vi "IMUOpen.vi"(4 "MagCal":bool, 5 "Accel Set":T5={"Data Rate"=enum."1.344 kHz", "Range"=0, "HPF Enable"=FALSE, "HPCF"=enum."00", "Sense Enable"=TRUE, "Accel Scale"={"Xscale"=1.0, "Yscale"=1.0, "Zscale"=1.0}, "Motion Thresh"=0.0} {"Range" items=["+/- 2 G", "+/- 4 G", "+/- 8 G", "+/- 16 G"]}, 6 "Mag Set":T2={"Data Rate"=enum."220 Hz", "Range"=1, "Sense Enable"=TRUE, "Mag Scale"={"Xscale"=1.0, "Yscale"=1.00987, "Zscale"=1.0}, "Mag Offset"={"Xzero"=0.181818, "Yzero"=-0.642644, "Zzero"=0.0}, "Anomaly Thresh"=0.646769, "Local Mag"=27.7309} {"Range" items=["+/- 130 uT"=1, "+/- 190 uT"=2, "+/- 250 uT"=3, "+/- 400 uT"=4, "+/- 470 uT"=5, "+/- 560 uT"=6, "+/- 810 uT"=7]}, 7 "Gyro Set":T6={"Data Rate"=enum."800 Hz", "Range"=0, "HPF Enable"=FALSE, "HPCF"=enum."0000", "Sense Enable"=TRUE} {"Range" items=["+/- 245 deg/sec", "+/- 500 deg/sec", "+/- 2000 deg/sec"]}, 8 "error in (no error)":errorcluster, 9 "Fast":bool=TRUE, 10 "CalSamples":i32=60, 11 "I2C Bus":T4) -> (0 "error out":errorcluster, 2 "Cal Result":T1, 3 "AdaIMUDevRef Out":T7={"DevStatus"={"status"=FALSE, "code"=0, "source"=""}, "Gyro Address"=0, "Gyro Range"=0, "Mean Rates"={"Xmo"=0.0, "Ymo"=0.0, "Zmo"=0.0}, "StdDev Rates"={"Xsdo"=0.0, "Ysdo"=0.0, "Zsdo"=0.0}, "Fast"=FALSE, "Reset"=FALSE, "Accel Address"=0, "Accel Range"=0, "Accel Scale"={"Xscale"=0.0, "Yscale"=0.0, "Zscale"=0.0}, "Mag Address"=0, "Mag Range"=0, "G Sense"=FALSE, "A Sense"=FALSE, "M Sense"=FALSE, "Accel Offset"={"Xzero"=0.0, "Yzero"=0.0, "Zzero"=0.0}, "Motion Thresh"=0.0, "Mag Scale"={"Xscale"=1.0, "Yscale"=1.0, "Zscale"=1.0}, "Mag Offset"={"Xzero"=1.0, "Yzero"=1.0, "Zzero"=1.0}, "I2C Bus"=enum."I2C On-Board", "Handle"=0, "Controller"=enum."Controller 1", "Anomaly Thresh"=0.0, "Local Mag"=0.0})   [LabVIEW 2014]
uses:
  IMUDevRef.ctl
  <vilib>/Rock Robotics/SystemInterfaces/i2clib/i2c_bus.ctl
  <vilib>/Rock Robotics/SystemInterfaces/Typedef/FPGA_TypedefDigitalModule.ctl
  <vilib>/Platform/TimedLoop/XDataNode/timing_clust.ctl
  <vilib>/Platform/TimedLoop/XDataNode/nitl_modes.ctl
  <vilib>/Platform/TimedLoop/XDataNode/wakeup.ctl
  <vilib>/Utility/file.llb/Write To Spreadsheet File (DBL).vi
  <vilib>/platform/TimedLoop/XDataNode/XDataNode.xnode
  <vilib>/Platform/TimedLoop/XDataNode/XDNodeRunTimeDep.lvlib
  <vilib>/Analysis/NI_AALBase.lvlib
panel:
  in  "Mag Set 2":T2={"Data Rate"=enum."220 Hz", "Range"=1, "Sense Enable"=TRUE, "Mag Scale"={"Xscale"=1.0, "Yscale"=1.0, "Zscale"=1.0}, "Mag Offset"={"Xzero"=0.0, "Yzero"=0.0, "Zzero"=0.0}, "Anomaly Thresh"=0.0, "Local Mag"=0.0} {"Range" items=["+/- 130 uT"=1, "+/- 190 uT"=2, "+/- 250 uT"=3, "+/- 400 uT"=4, "+/- 470 uT"=5, "+/- 560 uT"=6, "+/- 810 uT"=7]}
  out "XY Mag, Cal'd":cluster{dbl[], dbl[]}(graph)
  out "Anomaly Tol (uT)":dbl
  out "Local Magnitude (uT)":dbl
  out "Mid-Pnt":dbl
  out "Half-Range":dbl
  in  "Controller":T3
  out "Late?":bool
  in  "Period":i64=20
  out "Yaw":dbl(knob) scale=-180.0..180.0
  out "Pitch":dbl(knob) scale=-90.0..90.0
  out "Roll":dbl(knob) scale=-180.0..180.0
  in  "Reset":bool
  in  "Accel Set 2":T5={"Data Rate"=enum."1.344 kHz", "Range"=0, "HPF Enable"=FALSE, "HPCF"=enum."00", "Sense Enable"=TRUE, "Accel Scale"={"Xscale"=0.9852, "Yscale"=1.0101, "Zscale"=1.0101}, "Motion Thresh"=0.04} {"Range" items=["+/- 2 G", "+/- 4 G", "+/- 8 G", "+/- 16 G"]}
  in  "Gyro Set 2":T6={"Data Rate"=enum."800 Hz", "Range"=0, "HPF Enable"=FALSE, "HPCF"=enum."0000", "Sense Enable"=TRUE} {"Range" items=["+/- 245 deg/sec", "+/- 500 deg/sec", "+/- 2000 deg/sec"]}
  out "Xmagscale":dbl
  out "Ymagscale":dbl
  out "Ymagzero":dbl
  out "Xmagzero":dbl
  out "XY Mag":cluster{dbl[], dbl[]}(graph)
  out "stop loop":bool
  # "EXAMPLE MAGNETOMETER CAL PLOT - FOR REFERENCE"
  # "Magnetometer Cal Results"
  # "Use LM as Local Mag,\nwhich should be NOAA\nHorizontal Mag Intensity.\nUse AT as minimum\nAnomaly Threshold."
  # "Magnetometer Calibration Data Result\n\nLook for a constant radius circle - if not, repeat calibration.\n\nMagnetometer measurement error is generally classified into two categories, Hard Iron and Soft Iron effects.  Only Hard Iron effects\nare compensated here, as they appear more dominate.  Soft Iron effect compensation is a future improvement.  Performance is\nadequate as long as sources of Soft Iron distortion (non-magnetized Iron, Nickle, and Cobalt) are kept away from sensor\n(or vice versa).  If an ellipse is displayed, there is Soft Iron magnetic field interference.  Ensure the cal plot has equally sized X and Y\naxis ranges prior to visually inspecting the cal plot and making an ellipse determination.  If Soft Iron is detected, either relocate the\nIMU or discover and remove the offending material.  Run all motors and other actuators to verify that the Yaw output of the\nComplementary Filter is not significantly affected.  If so, it may be possible to relocate the IMU or shield the motor with\nmu-metal or similar.  Do not shield the IMU!"
  # "Reserved for future use."
  # "These controls/indicators are non-operational / they are here as example documentation only."
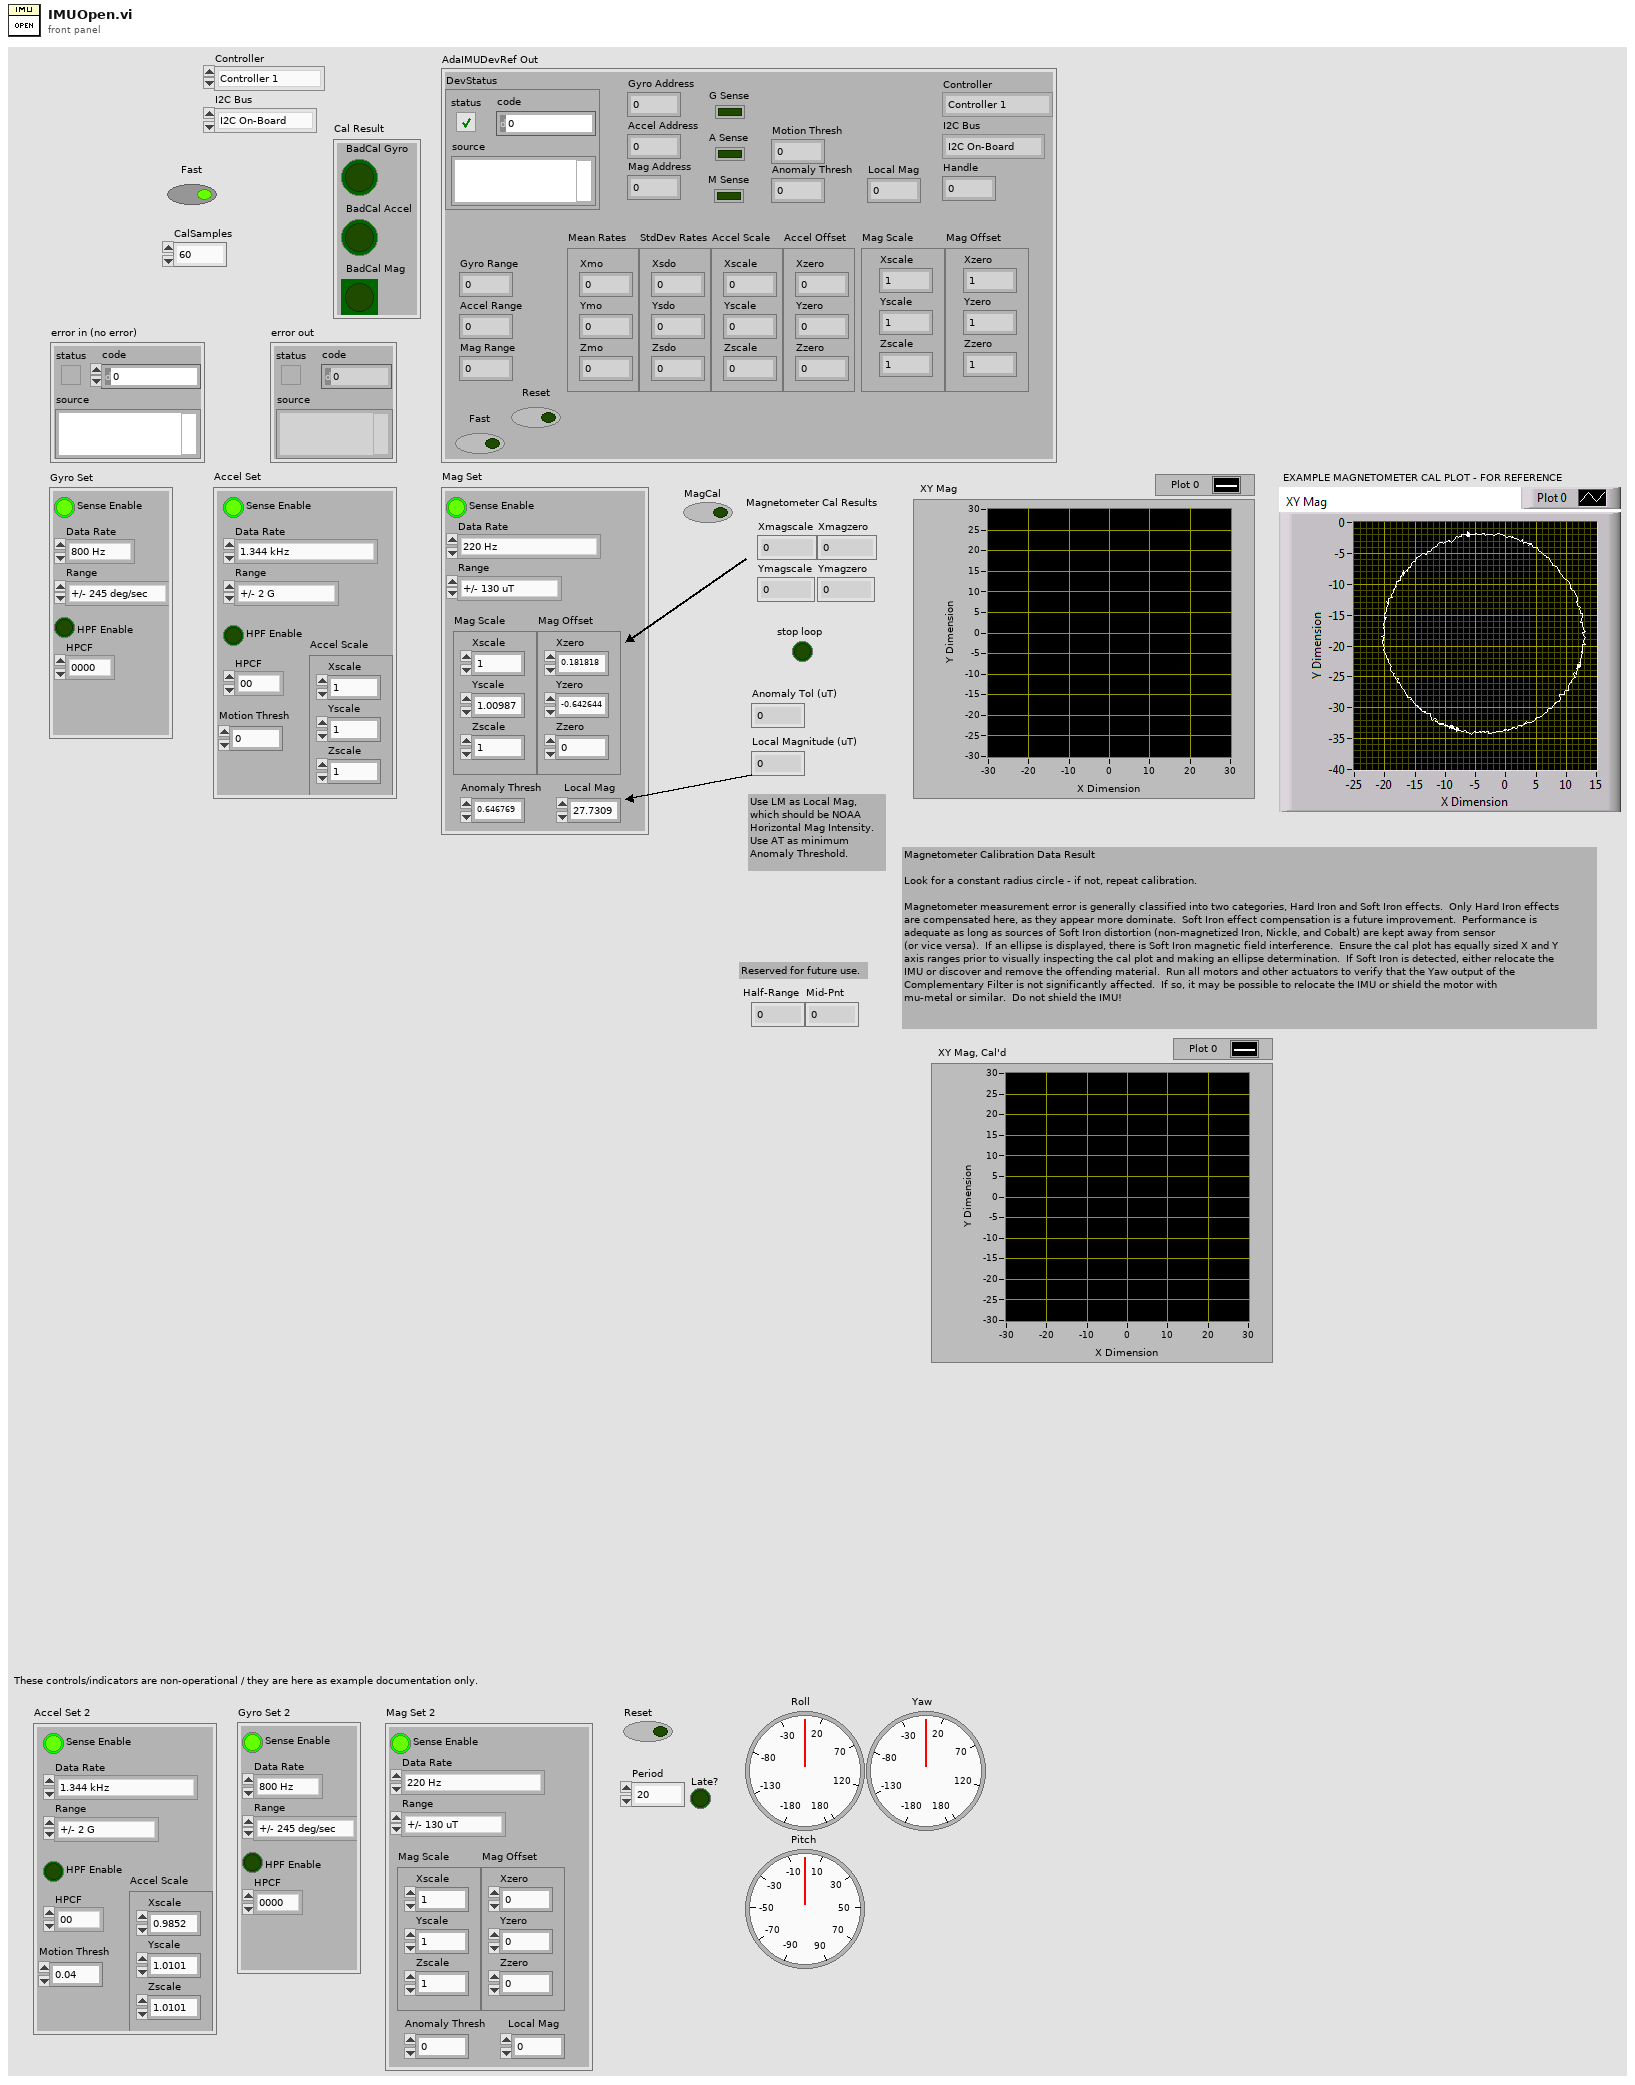
[diagram p1: front panel]
types:
  T1 = cluster{"BadCal Gyro":bool, "BadCal Accel":bool, "BadCal Mag":bool}
  T2 = cluster{"Data Rate":enum8{"0.75 Hz", "1.5 Hz", "3.0 Hz", "7.5 Hz", "15 Hz", "30 Hz", "75 Hz", "220 Hz"}, "Range":u8, "Sense Enable":bool, "Mag Scale":cluster{"Xscale":dbl, "Yscale":dbl, "Zscale":dbl}, "Mag Offset":cluster{"Xzero":dbl, "Yzero":dbl, "Zzero":dbl}, "Anomaly Thresh":dbl, "Local Mag":dbl}
  T3 = typedef "FPGA_TypedefDigitalModule.ctl" = enum16{"Controller 1"}
  T4 = typedef "i2c_bus.ctl" = enum16{"I2C On-Board", "I2C MXP", "Invalid"}
  T5 = cluster{"Data Rate":enum8{"Power-down mode", "1 Hz", "10 Hz", "25 Hz", "50 Hz", "100 Hz", "200 Hz", "400 Hz", "Low-power mode only", "1.344 kHz"}, "Range":u8, "HPF Enable":bool, "HPCF":enum8{"00", "01", "10", "11"}, "Sense Enable":bool, "Accel Scale":cluster{"Xscale":dbl, "Yscale":dbl, "Zscale":dbl}, "Motion Thresh":dbl}
  T6 = cluster{"Data Rate":enum8{"100 Hz", "200 Hz", "400 Hz", "800 Hz"}, "Range":u8, "HPF Enable":bool, "HPCF":enum8{"0000", "0001", "0010", "0011", "0100", "0101", "0110", "0111", "1000", "1001"}, "Sense Enable":bool}
  T7 = typedef "IMUDevRef.ctl" = cluster{"DevStatus":errorcluster, "Gyro Address":u8, "Gyro Range":u8, "Mean Rates":cluster{"Xmo":dbl, "Ymo":dbl, "Zmo":dbl}, "StdDev Rates":cluster{"Xsdo":dbl, "Ysdo":dbl, "Zsdo":dbl}, "Fast":bool, "Reset":bool, "Accel Address":u8, "Accel Range":u8, "Accel Scale":cluster{"Xscale":dbl, "Yscale":dbl, "Zscale":dbl}, "Mag Address":u8, "Mag Range":u8, "G Sense":bool, "A Sense":bool, "M Sense":bool, "Accel Offset":cluster{"Xzero":dbl, "Yzero":dbl, "Zzero":dbl}, "Motion Thresh":dbl, "Mag Scale":cluster{"Xscale":dbl, "Yscale":dbl, "Zscale":dbl}, "Mag Offset":cluster{"Xzero":dbl, "Yzero":dbl, "Zzero":dbl}, "I2C Bus":T4, "Handle":i32, "Controller":T3, "Anomaly Thresh":dbl, "Local Mag":dbl}
  T8 = enum8{"0000", "0001", "0010", "0011", "0100", "0101", "0110", "0111", "1000", "1001"}
  T9 = typedef "WPI_I2CDevRef.ctl" = cluster{"DevStatus":errorcluster, "Controller":T3, "Device Address":u8, "Handle":i32, "I2C Bus":T4}
  T10 = typedef "XDNodeRunTimeDep.lvlib/timing_clust.ctl" = cluster{"Expected End [f-1]":u64, "Actual End [f-1]":u64, "Finished Late? [f-1]":bool, "Expected End [i-1]":u64, "Actual End [i-1]":u64, "Finished Late? [i-1]":bool, "Expected Start [i]":u64, "Actual Start [i]":u64, "Expected Start [f]":u64, "Actual Start [f]":u64, "Source Name":string, "Structure Name":string, "Period":i64, "Deadline":i64, "Offset":i64, "Start":i64, "Priority":i32, "Timeout":i32, "Mode":T11, "Wakeup Reason":T12, "Error":errorcluster, "Source Type":string, "Secondary Source Type":string, "Global End Time":u64, "Global Start Time":u64, "Frame Duration":u64, "Iteration Duration":u64, "Assigned CPU":i32, "I/O Scan Engine Mode":u32}
  T11 = typedef "XDNodeRunTimeDep.lvlib/nitl_modes.ctl" = enum32{"No Change", "Process missed periods, maintain original phase", "Discard missed periods, maintain original phase", "Process missed periods, ignore original phase", "Discard missed periods, ignore original phase"}
  T12 = typedef "XDNodeRunTimeDep.lvlib/wakeup.ctl" = enum32{"Normal", "Aborted", "Asynchronous wakeup", "Timing source error", "Timed loop error", "Timeout"}
  T13 = typedef "Gyro.ctl" = cluster{"Xrate":dbl, "Yrate":dbl, "Zrate":dbl, "Xdeg":dbl, "Ydeg":dbl, "Zdeg":dbl, "dt":dbl}
  T14 = typedef "Accel.ctl" = cluster{"Xaccel":dbl, "Yaccel":dbl, "Zaccel":dbl, "Motion":bool, "Threshold":dbl, "FreeFall":bool}
  T15 = typedef "Mag.ctl" = cluster{"Xmag":dbl, "Ymag":dbl, "Zmag":dbl, "Anomaly":bool}
  T16 = enum8{"Power-down mode", "1 Hz", "10 Hz", "25 Hz", "50 Hz", "100 Hz", "200 Hz", "400 Hz", "Low-power mode only", "1.344 kHz"}
  T17 = cluster{"Xscale":dbl, "Yscale":dbl, "Zscale":dbl}
  T18 = enum8{"0.75 Hz", "1.5 Hz", "3.0 Hz", "7.5 Hz", "15 Hz", "30 Hz", "75 Hz", "220 Hz"}
  T19 = cluster{"Accel Zero.Zzero":dbl, "Accel Zero.Zzero 2":dbl, "Accel Zero.Zzero 3":dbl}
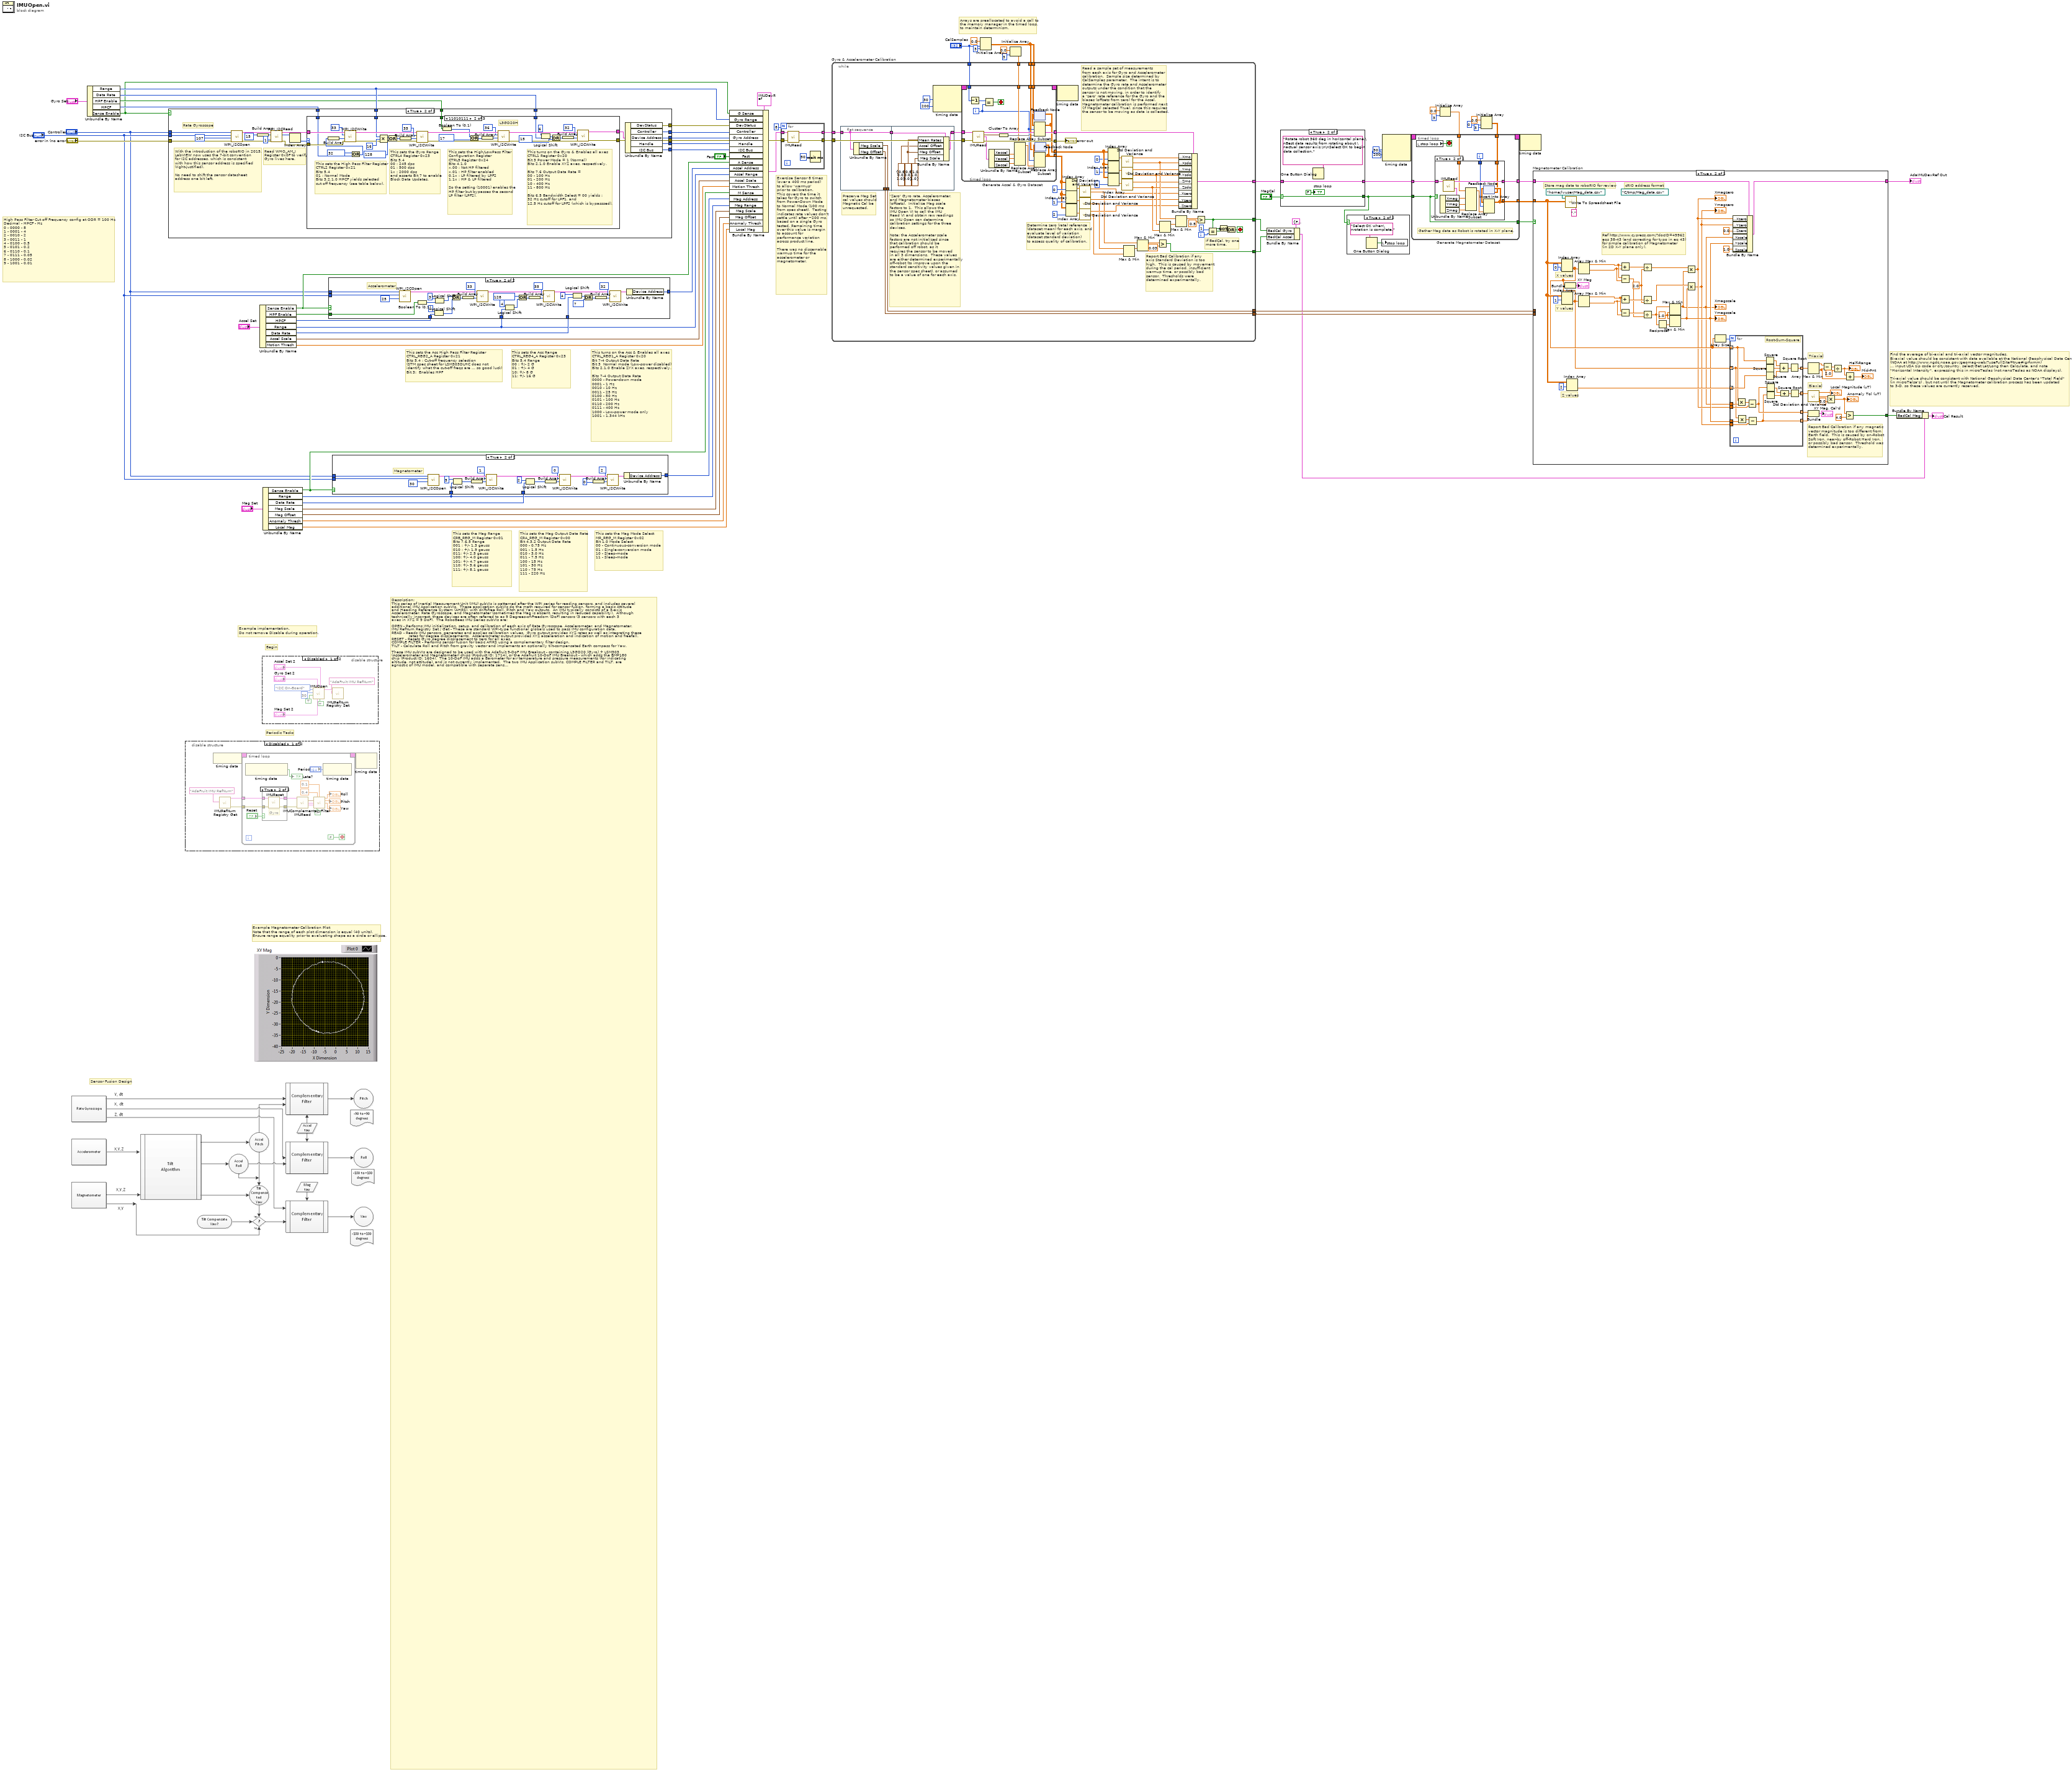
[diagram p0: block diagram]
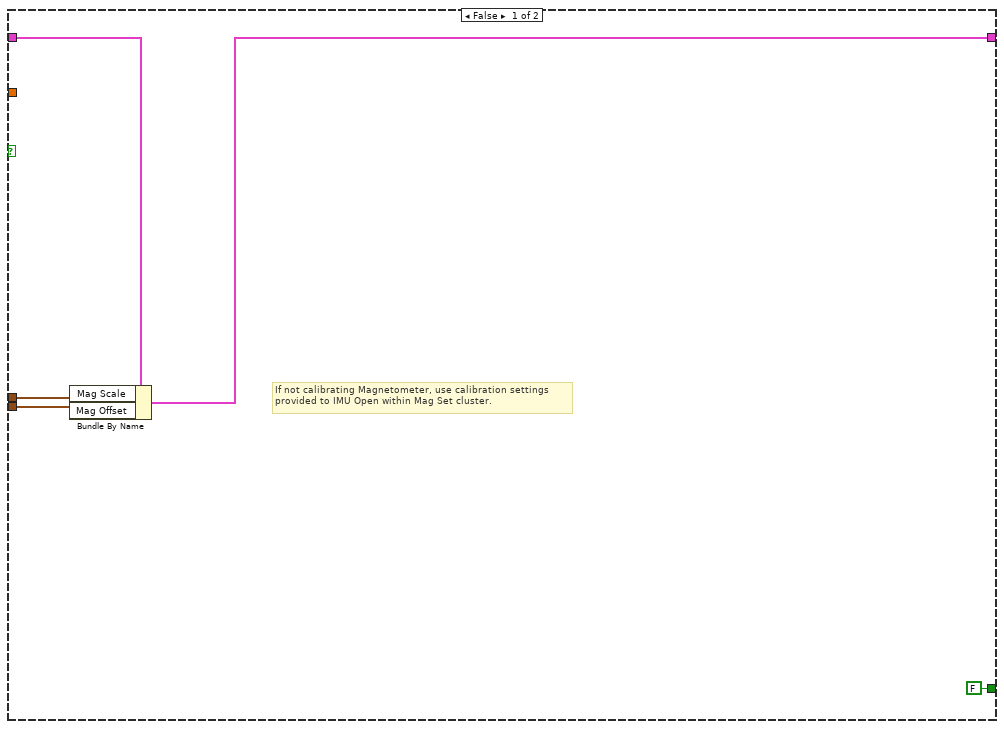
[diagram p2: hidden frame]
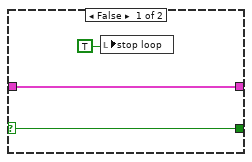
[diagram p5: hidden frame]
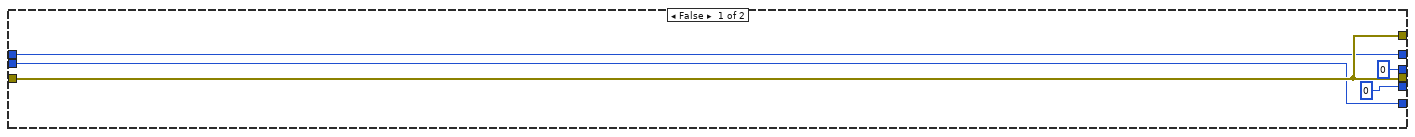
[diagram p9: hidden frame]
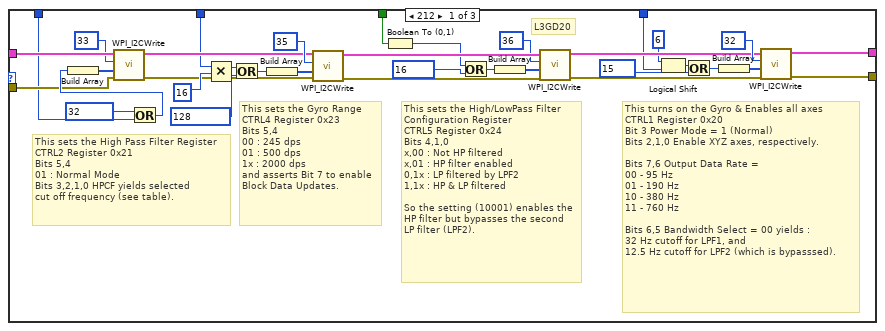
[diagram p10: hidden frame]
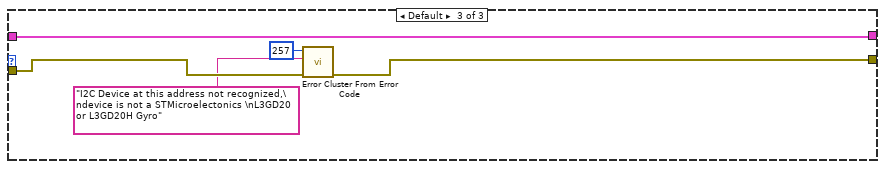
[diagram p11: hidden frame]
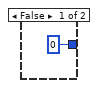
[diagram p12: hidden frame]
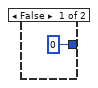
[diagram p13: hidden frame]
diagram:
  # "Find the average of bi-axial and tri-axial vector magnitudes.\nBi-axial value should be consistent with data available at the National Geophysical Data Center\n(NOAA at http://www.ngdc.noaa.gov/geomag-web/?useFullSite=true#igrfwmm)\n... input USA zip code or city/country, select Get Lat/Long then Calculate, and note\n\"Horizontal Intensity\", expressing this in microTeslas (not nanoTeslas as NOAA displays). \n\nTri-axial value should be consistent with National Geophysical Data Center's \"Total Field\"\n(in microTelsa's) , but not until the Magnetometer calibration process has been updated\nto 3-D, so these values are currently reserved."
  # "Arrays are preallocated to avoid a call to\nthe memory manager in the timed loop,\nto maintain determinism."
  # "Sensor Fusion Design"
  # "Example Magnetometer Calibration Plot\nNote that the range of each plot dimension is equal (40 units).\nEnsure range equality prior to evaluating shape as a circle or ellipse."
  # "Begin"
  # "Periodic Tasks"
  # "Example implementation.\nDo not remove Disable during operation."
  # "Description:\nThis series of Inertial Measurement Unit (IMU) subVIs is patterned after the WPI series for reading sensors, and includes several\nadditional IMU Application subVIs.  These application subVIs do the math required for sensor fusion, forming a basic Attitude\nand Heading Reference System (AHRS), with drift-free Roll, Pitch and Yaw outputs.  An IMU typically consists of a 3-axis \nAccelerometer, Rate Gyroscope, and Magnetometer (sometimes the Mag is absent, resulting in reduced capability).  Although\ntechnically incorrect, these devices are often referred to as 9 Degrees-of-Freedom (DoF) sensors (3 sensors with each 3\naxes in XYZ = 9 DoF).  The RoboBees IMU Series subVIs are:\n\nOPEN - Performs IMU initialization, setup, and calibration of each axis of Rate Gyroscope, Accelerometer, and Magnetometer.\nIMU RefNum Registry Set / Get - These are standard WPI-type functional globals used to pass IMU configuration data.\nREAD - Reads IMU sensors, generates and applies calibration values.  Gyro output provides XYZ rates as well as integrating these\n              rates for degree displacements.  Accelerometer output provides XYZ acceleration and indication of motion and freefall.\nRESET - Resets Gyro degree displacement to zero for all axes.\nCOMPLE FILTER - Performs sensor fusion for basic AHRS using a complementary filter design.\nTILT - Calculate Roll and Pitch from gravity vector and implements an optionally tilt-compensated Earth compass for Yaw.\n\nThese IMU subVIs are designed to be used with the Adafruit 9-DoF IMU Breakout - containing L3GD20 (Gyro) + LSM303 \n(Accelerometer and Magnetometer) chips (Product ID: 1714), or the Adafruit 10-DoF IMU Breakout - which adds the BMP180\nchip (Product ID: 1604).  The 10-DoF IMU adds a Barometer for air temperature and pressure measurements (for indicating\naltitude, not attitude), and is not currently implemented.  The two IMU Application subVIs, COMPLE FILTER and TILT, are\nagnostic of IMU model, and compatible with separate sensors, as long as all sensor axes are aligned properly.\n\nThe motivation to fusing these sensors is to combine their best properties and mitigate the worst properties of each.  The overall\nsensor fusion design is provided (to lower left) in block diagram form.  A major benefit is effective elimination of the drift inherent\nin the Rate Gyro when used alone.\n\nDesign:\nThe IMU OPEN subVI sets up each sensor based on the respective Set Cluster settings.  This includes setting the sensor range, output\ndata rate, enabling the High Pass Filter (Gyro and Accelerometer only), and selecting a High Pass Cut off Frequency.  Each sensor\ncan also be selectively enabled/disabled.  All sensors (except the Barometer), need to be enabled for a fully functional AHRS.  The\nIMU breakout board from Adafruit.com places all sensors on a common I2C bus for communication.  The sensor chip's I2C\nAddresses (in hex) and respective data sheets for I2C register references are:\n\nChip                      -  Sensor                - I2C Address  -  Data Sheet Reference\nLSM303DLHC      - Accelerometer   - 0x19               -  http://www.adafruit.com/datasheets/LSM303DLHC.PDF\nLSM303DLHC      - Magnetometer  - 0x1E               -  see above\nL3GD20(H)           - Rate Gyroscope - 0x6B               -  http://www.st.com/st-web-ui/static/active/en/resource/technical/document/\n                                                                                          datasheet/DM00036465.pdf\nBMP180               - Barometer           - 0x77               -  http://www.adafruit.com/datasheets/BST-BMP180-DS000-09.pdf\n\nNote: Adafruit modified both breakout board configurations in Oct of 2014 to upgrade the Gyro sensor from L3GD20 to L3GD20H\n(improved performance specifications).  This code should be compatible with each Gyro variant.  Guidance on the Gyro startup\nsequence is given in section 3.1 of ST MicroElectronics App Note AN4506 for L3GD20H : \nhttp://www.st.com/web/en/resource/technical/document/application_note/DM00119037.pdf\n\nAfter the sensors are set up, enabled sensors are turned on, IMU configuration data is loaded into an IMU Cluster, and sensor\ncalibration begins.\n\nCalibration:\nRaw readings from an IMU are not very useful until they are conditioned by carefully determined calibration parameters.\nSince reading the digital sensor values is a bit complicated, the IMU READ subVI is simply called by IMU OPEN to produce the raw\nmeasurement values used to characterize the sensor.  The calibration is only good for the range selected during the cal process.\n\nThe calibration process used here is determining the values 'm' and 'b' for the assumed linear sensor model Y=mX+b for each\nparameter/axis pair, where 'X' is the raw sensor reading, 'm' and 'b' are cal parameters, and 'Y' is the corrected sensor reading.\nThe sensor is 'exercised' eight times to allow the Gyro readings to reach steady-state, which improves the calibration.  With the\ndefault cal sample size of 60, the Gyro/Accelerometer cal process takes about 2.2 seconds, which is about 0.2 seconds longer\nthan the default cal time for the OPEN subVI for an analog Gyro.   The Gyro and Accelerometer cal is performed first\n(simultaneously), and the robot needs to be completely still during this time (as is required with an analog Gyro).  Since the cal\nis conducted within the OPEN subVI, and OPEN is generally placed in Begin (in FIRST Robotics) before the robot can move itself,\nthis requirement is easily fulfilled.  Care, however, must still be taken to ensure no external bumps occur during this cal.  This\ncode can actually detect if a physical disturbance occurred, and recalibrate automatically as a mitigation (no extra charge).\n\nRecalling the model Y=mX+b, for the IMU Gyro, 'm' is taken from the spec sheet as the gain (sensitivity) for each axis.  Value 'b',\nwhich is bias from zero, is determined by taking the statistical mean of a sample of Gyro rate measurements while the sensor is still.\n\nFor the Accelerometer, 'm' should be determined off-robot, as it requires the sensor to be moved in all 3 dimensions.  These values\nare either determined experimentally off-robot (to improve upon the standard sensitivity values given in the sensor spec sheet), or\nassumed to be a value of one for each axis.  To determine experimentally, find the maximum and minimum values of each axis as\nthey are rotated (slowly) through vertical.  The axis sensitivity is half of the signed difference between max and min.  Value 'b' is\ndetermined automatically by taking the statistical mean of a sample of Accelerometer measurements while the sensor is still.\n\nThe fun really begins with the Magnetometer calibration.  Proper Mag cal requires the sensor to be rotated in all 3 dimensions, but\nunlike the Accelerometer, the Mag must be rotated with the rest of the robot to account for how the robot itself disturbs the Earth's\nmagnetic field (this is a lot easier when the Mag sensor is installed in a smart phone.).  Since one typically would not have available\na 3-axis non-ferrous robot gimbal, the cal process is designed to support a 2-D calibration in the X-Y (horizontal) plane only.\n\nIn another departure from the Gyro/Accel cal, sample data from the Mag must be taken as the robot is moving.  This process is\noptional to allow the 'm' and 'b' Mag cal parameters to be determined during final testing, and then loaded into the Mag Set Cluster\nfor operations (i.e. competition).  If selected, the Mag cal process first instructs you to begin rotating the robot (manually) with a \npop-up dialog box.  Selecting OK initiates data collection, and provides a second dialog box to allow you to signal when you've \ncompleted a 360 degree rotation.  \n\nOnce complete, the X and Y axis 'm' and 'b' parameters are calculated and displayed on the IMU OPEN Front Panel as 'scale' and\n'zero', respectively.  An XY graph of the data is also provided to allow visual inspection of the cal result - look for a nicely shaped\ncircle (see example at left), if not, repeat the cal.  If you like the plot, load the X and Y axis scale and zero parameters into the Mag\nSet Cluster, retain the default scale (1) and zero (0) values for the Mag Z axis, and turn off Mag cal by deasserting MagCal.\n\nMagnetometer measurement error is generally classified into two categories, Hard Iron and Soft Iron effects.  Only Hard Iron effects\nare compensated here, as they appear to dominate.  Soft Iron effect compensation is a future improvement.  Performance is\nadequate as long as sources of Soft Iron distortion (non-magnetized Iron, Nickle, and Cobalt) are kept away from sensor\n(or vice versa).  If an ellipse is displayed, there is Soft Iron magnetic field interference.  Ensure the cal plot has equally sized X and Y\naxis ranges prior to visually inspecting the cal plot and making an ellipse determination.  If Soft Iron is detected, either relocate the\nIMU or discover and remove the offending material.  Run all motors and other actuators to verify that the Yaw output of the\nComplementary Filter is not significantly affected.  If so, it may be possible to relocate the IMU or shield the motor with\nmu-metal or similar.  Do not shield the IMU!\n\nInputs:\nDIO MODULE - Digital Module designation.\nCALSAMPLES - Number of samples taken for Gyro and Accelerometer calibration process.\nFAST - Boolean, if True, bypasses sensor data ready status verification in the interest of faster IMU Read operations.\n             Setting this to False will force each sensor to verify that data is ready prior to an IMU Read.\nMAGCAL - Boolean, if True, activates the Magnetometer calibration process within IMU OPEN.\n                    Setting this to False skips the Mag cal process, applying cal parameters defined in the Mag Set Cluster during IMU Read.\nGYRO SET -\n     SENSE ENABLE - Enables the Gyro Sensor when True, allowing OPEN IMU to set up and turn on the Gyro, and READ IMU to read. \n                                   Setting this to False speeds up the IMU READ operation, should this sensor not be required.\n     DATA RATE - Sets the sensor output data rate in Hertz. \n     RANGE - Sets the sensor range, in degrees / second.\n     HPF ENABLE - Enables the Gyro High Pass Filter when True. \n     HPCF - Sets the High Pass Cut off Frequency.  Values are specific enumerated binary nybbles that correspond to cut off\n                   frequencies in Hertz.  See Table (near code) for selections at 100 Hz data rate.  See spec sheet for additional detail.\nACCEL SET - \n     SENSE ENABLE -  Enables the Accel Sensor when True, allowing OPEN IMU to set up and turn on the Accel, and READ IMU to read.\n                                    Setting this to False speeds up the IMU READ operation, should this sensor not be required. \n     DATA RATE - Sets the sensor output data rate in Hertz.\n     RANGE - Sets the sensor range, in G's (1 G is ~ 9.805 meters / second^2).  The Earth's gravity field is, well, about 1 G at sea level.\n     HPF ENABLE - Enables the Accelerometer High Pass Filter when True. \n     HPCF - Sets the High Pass Cut off Frequency.  Values are specific enumerated bit pairs that correspond to cut off frequencies in\n                   Hertz.  Spec sheet does not define to what cut off frequencies these settings correspond.  Suggest experiment.\n     ACCEL SCALE - Multiplier value for each axis to correct for imperfection in spec sheet cal factors. \n     MOTION THRESH - Threshold value used to signal the detection of Motion or Free Fall, specified in G's. \nMAG SET - \n     SENSE ENABLE -  Enables the Mag Sensor when True, allowing OPEN IMU to set up and turn on the Mag, and READ IMU to read.\n                                   Setting this to False speeds up the IMU READ operation, should this sensor not be required. \n     DATA RATE - Sets the sensor output data rate in Hertz.\n     RANGE - Sets the sensor range, in microTesla's (1 uT = 0.01 Gauss).  The Earth's magnetic field (magnitude) is about 0.5 Gauss,\n                     or ~50 uT, with both horizontal (North and East) and vertical (Down) components that change with locale (and time). \n     MAG SCALE -  Multiplier value to correct raw Magnetometer reading to calibrated value.  Calculated by the Mag cal process.\n     MAG OFFSET - Offset value to correct raw Magnetometer reading to calibrated value.  Calculated by the Mag cal process.\n     ANOMALY THRESH - Threshold value used to signal the detection of a magnetic anomoly, i.e. a disturbance in the Earth field,\n                                            specified in uTeslas.\n     LOCAL MAG - Bi-axial horizontal vector magnitude of local Earth's magnetic field, specified in uTeslas.\n     \nOutputs:\nADAIMUDEVREF OUT - Device Reference containing IMU configuration data. \nBADCAL GYRO - Boolean, if True, indicates excessive variation in sample data set.  Likely Gyro moved during cal process.  If True,\n                              Gyro cal process will automatically repeat one additional time in an attempt to recover.\n                              If False, sample data set variation low enough to indicate Gyro was still during cal, and zero-rate mean is trusted. \nBADCAL ACCEL - Boolean, if True, indicates excessive variation in sample data set.  Likely Accel moved during cal process.\n                              If False, sample data set variation low enough to indicate Accel was still during cal, and mean is trusted as the bias.\nBADCAL MAG - Boolean, if True, indicates excessive variation in the magnetic field as measured during calibration.  Possible causes\n                             are nearby hard iron off-robot, soft iron on-robot, or poor rotation during calibration.\n\nFuture Improvements:\nBarometer, move freefall into interrupt/DIO, DCM/Kalman filter, Soft Iron Calibration, 3D cal, Auto ranging, FPGA integration,\nFuse Mag-based Yaw with differential encoders to correct for external-to-robot ferrous sources, SPI interface for faster read response,\nCal status VI\n\nVI Properties:\nExecution Reentrancy is set to Non Reentrant Execution\n\nImplementation:\nCode as per example on upper left.  Experimentally determine values for Accelerometer scale as described in above section on\ncalibration, and load into the Accel Set Cluster (or default to one).  Set appropriate ranges, fastest data rates (if polling), and enable\neach sensor. Install sensor on robot and initially set MagCal to True.  Determine Mag cal parameters as described above and load\nthese values into Mag Set Cluster.  Set MagCal to False to skip future Mag cals.\n\nMagnetic Anomalies are detected during IMU READ operation by comparing the root-sum-square of the X-Y axes to the horizontal\nmagnitude of the local Earth field, based on two settings which must be specified in the IMU OPEN Mag Set Cluster.  The first setting\nis LOCAL MAG, representing the biaxial horizontal vector magnitude of the Earth's local magnetic field.  This can be found from data\navailable at the National Geophysical Data Center, part of the National Oceanic and Atmospheric Administration (NOAA) at :\n\nhttp://www.ngdc.noaa.gov/geomag-web/?useFullSite=true#igrfwmm\n\nTo find the value for LOCAL MAG, input USA zip code or city/country, select Get Lat/Long then Calculate, and use the \"Horizontal Intensity\"\nvalue for Local Mag, expressing this in uTeslas (not nTeslas as NOAA displays), or use the calculated value \"Local Magnitude (uT)\" produced\nby this VI (under Magnetometer Cal Results).  The second setting is ANOMALY THRESH, also specified in the Mag Set Cluster, and is used as\ntolerance for the comparison.  Set to a value at least as large as \"Anomaly Tol (uT)\", also produced by this VI.  Based on these settings,\nIMU READ produces a Boolean Magnetic Anomaly indication that can be used to determine when the Magnetometer is reading more than\nthe Earth's field. In this situation, the Yaw output of the sensor fusion Complementary Filter should not be trusted to be accurate.\n\nThe anomaly threshold can be increased above the value reported as Anomaly Tol (uT) to avoid false positive indications, but this is at the\nexpense of reduced sensitivity to actual magnetic anomalies.  Ideally, detection of a Magnetic Anomaly should occur before the Yaw\nreading is substantially affected.  This may be difficult to achieve without very careful calibration of the Mag, and careful selection of the\nanomaly threshold.  \n \nThe Mag cal values are strongly a function of where the sensor is located on the robot, and what is installed nearby, so it's important\nto recalibrate fairly often, certainly after relocating the sensor, and again after the robot is completely assembled.  Be sure you actuate\nall motors and mechanisms to test for interaction with the Yaw indication, which uses the Mag.  Be aware that another robot that\ncomes close to the Magnetometer might disturb the local magnetic field enough to cause error in Yaw - the solution to this difficulty\nis left to the enterprising student of sensor fusion.\n\nEnabling the Gyro and Accelerometer High Pass Filters (HPF) can have a deleterious effect on dynamic response, as they can\nintroduce lag.  HPFs default to off, but advanced control system designers may find them useful.  Experiment cautiously.\n\nThe Accelerometer senses both gravitation and accelerating movement (study Einstein's principle of Equivalence).  Roll and Pitch may be\naffected by movement, as will Yaw should Tilt-Compensation be enabled (this is selected with the Comple Filter subVI).\n\nConfiguring these IMU subVIs per the example creates a simple Attitude and Heading Reference System (AHRS).  The range of Pitch/\nRoll/Yaw values are constrained in range, however, as follows:  Pitch range is -90<P<+90, Roll range is -180<R<+180, and Yaw range\nis -180<Y<+180.  Although over-rotating Pitch and Yaw beyond their range will result in erroneous readings, this should be an\nadequate operating range for most robot body applications.  These range constraints may or may not be adequate for an actuator\nor mechanism.  Yaw is a bit different ...  North is 0 degrees, and East/West  is -90/+90 deg, respectively.  South is both -180 and +180\ndeg, as these values are congruent.  It is ok to over-rotate Yaw, as this portion of the Complementary Filter is designed with logic to\nsmoothly transition across the +/-180 degree discontinuity (auto-wrap).\n \nIt is important to note that while the P/R/Y values are constrained, the Gyro displacement values in X/Y/Z are not.  Gyro deg outputs\nfrom the IMU READ subVI will wind (not wrap) - i.e. they will continue to count above/below 360 degrees.  Use the LabVIEW\nQuotient & Remainder (modulus) function to convert these outputs to a wrapping behavior, if desired. \n\nImplementation considerations for IMU Read:\nThis design performs numerical integration off-FPGA for the Digital Gyro (unlike the Analog Gyro subVIs, which typically utilize\nthe FPGA to perform accumulation for superior speed resulting in less integration error).   Testing indicates this off-FPGA\napproach may be adequate for FRC application, however, it is important to ensure the code runs without any timing issues.\nThis is why a Timed Loop is recommended for the IMU Read within Periodic Tasks (executes at a higher priority).  Non-uniformity\nin read iteration is mitigated by design, as each dt is uniquely calculated by time stamping each read event.  This means that while\nsome variation in timing can be tolerated (the occasional late iteration), excessively long durations (periods) between successive\nreads will fail to capture the actual rate profile as it changes resulting in integration error.  \n\nIn short, use a Timed Loop structure to iterate IMU READs, and set the loop period for a relatively fast iteration (<75 ms).  Shorter\nperiods provide improved accuracy of degree displacements, however setting this too short can impact the execution of your\nremaining code (especially when using Timed Loops).  One way of determining an optimized period is to set it while monitoring\nthe \"Finished Late?\" Loop parameter, ensuring this value stays False.   It helps if the CPU Utilization remains low (<75%), which\ncan be monitored with the RT Get CPU Loads subVI (Real Time menu).  Study LabVIEW determinism for additional insight.\n\n----- RoboBees FRC Team 836! -----  You too can conquer inertia!! ... consider a career in STEM!"
  # "This sets the Mag Mode Select\nMR_REG_M Register 0x02\nBit 1,0 Mode Select\n00 - Continuous-conversion mode \n01 - Single-conversion mode\n10 - Sleep-mode\n11 - Sleep-mode"
  # "This sets the Mag Output Data Rate\nCRA_REG_M Register 0x00\nBit 4,3,2 Output Data Rate\n000 - 0.75 Hz \n001 - 1.5 Hz \n010 - 3.0 Hz\n011 - 7.5 Hz\n100 - 15 Hz\n101 - 30 Hz\n110 - 75 Hz\n111 - 220 Hz"
  # "This sets the Mag Range\nCRB_REG_M Register 0x01\nBits 7,6,5 Range\n001 : +/- 1.3 gauss\n010 : +/- 1.9 gauss\n011: +/- 2.5 gauss\n100: +/- 4.0 gauss\n101: +/- 4.7 gauss\n110: +/- 5.6 gauss\n111: +/- 8.1 gauss"
  # "This sets the Acc Range\nCTRL_REG4_A Register 0x23\nBits 5,4 Range\n00 : +/- 2 G\n01 : +/- 4 G\n10: +/- 8 G\n11: +/- 16 G"
  # "This turns on the Acc & Enables all axes\nCTRL_REG1_A Register 0x20\nBit 7-4 Output Data Rate\nBit 3  Normal mode (Low-power disabled)\nBits 2,1,0 Enable ZYX axes, respectively.\n\nBits 7-4 Output Data Rate \n0000 - Power-down mode\n0001 - 1 Hz \n0010 - 10 Hz\n0011 - 25 Hz\n0100 - 50 Hz\n0101 - 100 Hz\n0110 - 200 Hz\n0111 - 400 Hz\n1000 - Low-power mode only\n1001 - 1.344 kHz"
  # "This sets the Acc High Pass Filter Register\nCTRL_REG2_A Register 0x21\nBits 5,4 : Cut-off frequency selection\n(STM spec sheet for LSM303DLHC does not\nidentify what the cut-off freqs are ... so good luck)\nBit 3:  Enables HPF"
  # "High Pass Filter Cut off Frequency config at ODR = 100 Hz\nDecimal\t-\tHPCF\t-\tHz\n0\t-\t0000\t-\t8\n1\t-\t0001\t-\t4\n2\t-\t0010\t-\t2\n3\t-\t0011\t-\t1\n4\t-\t0100\t-\t0.5\n5\t-\t0101\t- 0.2\n6\t-\t0110\t-\t0.1\n7\t-\t0111\t-\t0.05\n8\t-\t1000\t-\t0.02\n9\t-\t1001\t-\t0.01"
  # "Exercise Sensor 8 times\n(over a 400 ms period)\nto allow 'warmup'\nprior to calibration.\nThis covers the time it\ntakes for Gyro to switch\nfrom Power-Down Mode\nto Normal Mode (100 ms\nfrom spec sheet).  Testing\nindicates rate values don't\nsettle until after ~200 ms,\nbased on a single Gyro\ntested. Remaining time\nover this value is margin\nto account for\nperformance variation\nacross product line.\n\nThere was no discernable\nwarmup time for the\naccelerometer or\nmagnetometer."
  n1 = Unbundle By Name("Gyro Set") -> ("Range"=w63:u8, "Data Rate"=w62:enum8{"100 Hz", "200 Hz", "400 Hz", "800 Hz"}, "HPF Enable"=w61:bool, "HPCF"=w60:T8, "Sense Enable"=w53:bool)
  n2 = case shown="True" w53 {
    tunnel: "error in (no error)" -> [w78 w102]
    tunnel: [w78 w91] -> w71
    tunnel: [u8 0 ("Device Address") w90] -> w70
    tunnel: [w78 w89] -> w48
    tunnel: w63 -> [_ w88]
    tunnel: w62 -> [_ w87]
    tunnel: w61 -> [_ w86]
    tunnel: w60 -> [_ w85]
    tunnel: "I2C Bus" -> [w75 w84]
    tunnel: [0 ("Handle") w83] -> w43
    tunnel: [w75 w82] -> w44
    tunnel: "Controller" -> [w74 w80]
    tunnel: [w74 w81] -> w42
    frame False {
    }
    frame True {
      # "Rate Gyroscope"
      # "Read WHO_AM_I \nRegister 0x0F to verify\nGyro lives here."
      # "With the introduction of the roboRIO in 2015,\nLabVIEW now uses the 7-bit convention\nfor I2C addresses, which is consistent\nwith how this sensor address is specified\n(right-justified).\n\nNo need to shift the sensor datasheet\naddress one bit left."
      n3 = call <vilib>:"WPI_I2COpen.vi"("error in"=w102, "Device Address"=u8 107 ("Data To Send"), "I2C Bus"=w84, "Controller"=w80) -> ("error out"=w98:errorcluster, "I2CDevRef"=w93:T9)  [unwired: 6 in]
      n4 = Build Array(u8 15 ("Data To Send")) -> (w100:u8[])
      n5 = call <vilib>:"WPI_I2CRead.vi"("error in (no error)"=w98, "I2CBytesToRead"=u8 1, "I2CRegister"=w100, "I2CDevRef"=w93) -> ("error out"=w95:errorcluster, "Data Out"=w97:u8[], "I2CDevRef"=w94:T9)  [unwired: 5 in]
      n6 = Index Array(array=w97) -> (element=w96:u8)  [unwired: 1 in]
      n7 = case shown="11010111" w96 {
        tunnel: [w137 w172 w177] -> w92
        tunnel: [w136 w171 w173] -> w89
        tunnel: w94 -> [w135 w170 w177]
        tunnel: w95 -> [w120 w156 w176]
        tunnel: w88 -> [w116 w152 _]
        tunnel: w85 -> [w115 w151 _]
        tunnel: w86 -> [w110 w146 _]
        tunnel: w87 -> [w106 w140 _]
        frame 212 {
          # "L3GD20"
          # "This sets the High Pass Filter Register\nCTRL2 Register 0x21\nBits 5,4\n01 : Normal Mode\nBits 3,2,1,0 HPCF yields selected\ncut off frequency (see table)."
          # "This sets the High/LowPass Filter\nConfiguration Register\nCTRL5 Register 0x24\nBits 4,1,0  \nx,00 : Not HP filtered\nx,01 : HP filter enabled\n0,1x : LP filtered by LPF2\n1,1x : HP & LP filtered\n\nSo the setting (10001) enables the\nHP filter but bypasses the second\nLP filter (LPF2)."
          # "This sets the Gyro Range\nCTRL4 Register 0x23\nBits 5,4\n00 : 245 dps\n01 : 500 dps\n1x : 2000 dps\nand asserts Bit 7 to enable Block Data Updates."
          # "This turns on the Gyro & Enables all axes\nCTRL1 Register 0x20\nBit 3 Power Mode = 1 (Normal)\nBits 2,1,0 Enable XYZ axes, respectively.\n\nBits 7,6 Output Data Rate = \n00 - 95 Hz\n01 - 190 Hz \n10 - 380 Hz\n11 - 760 Hz\n\nBits 6,5 Bandwidth Select = 00 yields : \n32 Hz cutoff for LPF1, and\n12.5 Hz cutoff for LPF2 (which is bypasssed)."
          n8 = Or(x=u8 32 ("Data To Send"), y=w115) -> (x .or. y?=w125:u8)
          n9 = Build Array(w125) -> (w128:u8[])
          n10 = call <vilib>:"WPI_I2CWrite.vi"("error in (no error)"=w120, "I2CDataToSend"=w128, "I2CRegister"=u8 33 ("Data To Send"), "I2CDevRef"=w135) -> ("error out"=w119:errorcluster, "I2CDevRef"=w127:T9)  [unwired: 6 in]
          n11 = Multiply(x=w116, y=u8 16) -> (x*y=w114:u8)
          n12 = Or(x=w114, y=u8 128 ("Data To Send")) -> (x .or. y?=w113:u8)
          n13 = Build Array(w113) -> (w132:u8[])
          n14 = call <vilib>:"WPI_I2CWrite.vi"("error in (no error)"=w119, "I2CDataToSend"=w132, "I2CRegister"=u8 35 ("Data To Send"), "I2CDevRef"=w127) -> ("error out"=w118:errorcluster, "I2CDevRef"=w124:T9)  [unwired: 6 in]
          n15 = Boolean To (0,1)(Boolean=w110) -> (0, 1=w104:i16)
          n16 = Or(x=w104, y=u8 16 ("Data To Send")) -> (x .or. y?=w112:i16)
          n17 = Build Array(w112) -> (w121:i16[])
          n18 = call <vilib>:"WPI_I2CWrite.vi"("error in (no error)"=w118, "I2CDataToSend"=w121, "I2CRegister"=u8 36 ("Data To Send"), "I2CDevRef"=w124) -> ("error out"=w117:errorcluster, "I2CDevRef"=w123:T9)  [unwired: 6 in]
          n19 = Logical Shift(y=i16 6, x=w106) -> (x << y=w107:u32)
          n20 = Or(x=w107, y=u8 15 ("Data To Send")) -> (x .or. y?=w109:u32)
          n21 = Build Array(w109) -> (w133:u32[])
          n22 = call <vilib>:"WPI_I2CWrite.vi"("error in (no error)"=w117, "I2CDataToSend"=w133, "I2CRegister"=u8 32 ("Data To Send"), "I2CDevRef"=w123) -> ("error out"=w136:errorcluster, "I2CDevRef"=w137:T9)  [unwired: 6 in]
        }
        frame 215 {
          # "L3GD20H"
          # "This sets the High Pass Filter Register\nCTRL2 Register 0x21\nBits 5,4\n01 : Normal Mode\nBits 3,2,1,0 HPCF yields selected\ncut off frequency (see table below)."
          # "This sets the High/LowPass Filter\nConfiguration Register\nCTRL5 Register 0x24\nBits 4,1,0  \nx,00 : Not HP filtered\nx,01 : HP filter enabled\n0,1x : LP filtered by LPF2\n1,1x : HP & LP filtered\n\nSo the setting (10001) enables the\nHP filter but bypasses the second\nLP filter (LPF2)."
          # "This sets the Gyro Range\nCTRL4 Register 0x23\nBits 5,4\n00 : 245 dps\n01 : 500 dps\n1x : 2000 dps\nand asserts Bit 7 to enable Block Data Updates."
          # "This turns on the Gyro & Enables all axes\nCTRL1 Register 0x20\nBit 3 Power Mode = 1 (Normal)\nBits 2,1,0 Enable XYZ axes, respectively.\n\nBits 7,6 Output Data Rate = \n00 - 100 Hz\n01 - 200 Hz \n10 - 400 Hz\n11 - 800 Hz\n\nBits 6,5 Bandwidth Select = 00 yields : \n32 Hz cutoff for LPF1, and\n12.5 Hz cutoff for LPF2 (which is bypasssed)."
          n23 = Or(x=u8 32 ("Data To Send"), y=w151) -> (x .or. y?=w161:u8)
          n24 = Build Array(w161) -> (w164:u8[])
          n25 = call <vilib>:"WPI_I2CWrite.vi"("error in (no error)"=w156, "I2CDataToSend"=w164, "I2CRegister"=u8 33 ("Data To Send"), "I2CDevRef"=w170) -> ("error out"=w155:errorcluster, "I2CDevRef"=w163:T9)  [unwired: 6 out]
          n26 = Multiply(x=w152, y=u8 16) -> (x*y=w150:u8)
          n27 = Or(x=w150, y=u8 128 ("Data To Send")) -> (x .or. y?=w149:u8)
          n28 = Build Array(w149) -> (w168:u8[])
          n29 = call <vilib>:"WPI_I2CWrite.vi"("error in (no error)"=w155, "I2CDataToSend"=w168, "I2CRegister"=u8 35 ("Data To Send"), "I2CDevRef"=w163) -> ("error out"=w154:errorcluster, "I2CDevRef"=w160:T9)  [unwired: 6 out]
          n30 = Boolean To (0,1)(Boolean=w146) -> (0, 1=w147:i16)
          n31 = Or(x=w147, y=u8 17 ("Data To Send")) -> (x .or. y?=w145:i16)
          n32 = Build Array(w145) -> (w157:i16[])
          n33 = call <vilib>:"WPI_I2CWrite.vi"("error in (no error)"=w154, "I2CDataToSend"=w157, "I2CRegister"=u8 36 ("Data To Send"), "I2CDevRef"=w160) -> ("error out"=w153:errorcluster, "I2CDevRef"=w159:T9)  [unwired: 6 out]
          n34 = Logical Shift(y=i16 6, x=w140) -> (x << y=w142:u32)
          n35 = Or(x=w142, y=u8 15 ("Data To Send")) -> (x .or. y?=w138:u32)
          n36 = Build Array(w138) -> (w139:u32[])
          n37 = call <vilib>:"WPI_I2CWrite.vi"("error in (no error)"=w153, "I2CDataToSend"=w139, "I2CRegister"=u8 32 ("Data To Send"), "I2CDevRef"=w159) -> ("error out"=w171:errorcluster, "I2CDevRef"=w172:T9)  [unwired: 6 out]
        }
        frame Default {
          n38 = call <vilib>:"Error Cluster From Error Code.vi"("error in (no error)"=w176, "error message (\"\")"="I2C Device at this address not recognized,\ndevice is not a STMicroelectonics \nL3GD20 or L3GD20H Gyro" ("error message (\"\")"), "error code (0)"=257) -> ("error out"=w173:errorcluster)  [unwired: 6 in]
        }
      }
      n39 = Unbundle By Name(w92) -> ("DevStatus"=w91:errorcluster, "Controller"=w81:T3, "Device Address"=w90:u8, "Handle"=w83:i32, "I2C Bus"=w82:T4)
    }
  }
  n40 = disable-structure shown="Disabled" {
    frame Disabled {
      n41 = node-c288() -> (w182:T10)
      n42 = call "IMURefNum Registry Get.vi"("refnum name"="AdaFruit IMU RefNum") -> ("error out"=w178:errorcluster, "AdaIMUDevRef Out"=w179:T7)  [unwired: 9 in]
      n43 = timed-loop {
        tunnel: w179 -> [w196]
        tunnel: w178 -> [w195]
        timing: w182 -> [_]
        timing-out: [_] -> w181
        stop <- FALSE stop-if-true
        n44 = node-c288() -> (→"Late?":bool)  [unwired: 1 in]
        n45 = case shown="True" "Reset" {
          tunnel: w196 -> [w206 w210]
          tunnel: [w206 w209] -> w198
          tunnel: [w205 w208] -> w197
          tunnel: w195 -> [w205 w207]
          frame False {
          }
          frame True {
            # "Gyro"
            n46 = call "IMUReset.vi"("error in (no error)"=w207, "AdaIMUDevRef"=w210) -> ("error out"=w208:errorcluster, "AdaIMUDevRef Out"=w209:T7)  [unwired: 8 in]
          }
        }
        n47 = call "IMURead.vi"("AdaIMUDevRef"=w198, "error in"=w197) -> ("Gyro"=w193:T13, "Accel"=w192:T14, "Mag"=w191:T15)  [unwired: 9 in, 2 out]
        n48 = call "IMUComplementaryFilter.vi"("tau acc"=0.4, "tau mag"=0.1, "Gyro"=w193, "Accel"=w192, "Mag"=w191, "Tilt Comp (Yaw)"=FALSE) -> ("Roll"=→"Roll":dbl, "Pitch"=→"Pitch":dbl, "Yaw"=→"Yaw":dbl)  [unwired: 6 in, 1 out]
        n49 = node-c288("Period") -> ()  [unwired: 1 out]
      }
      n50 = node-c288(w181) -> ()  [unwired: 1 out]
    }
    frame Enabled {
    }
  }
  n51 = Unbundle By Name("Accel Set") -> ("Sense Enable"=w51:bool, "HPF Enable"=w67:bool, "HPCF"=w66:enum8{"00", "01", "10", "11"}, "Range"=w58:u8, "Data Rate"=w65:T16, "Accel Scale"=w59:T17, "Motion Thresh"=w56:dbl)
  n52 = disable-structure shown="Disabled" {
    frame Disabled {
      n53 = call "IMUOpen.vi"("MagCal"=TRUE, "Accel Set"="Accel Set 2", "Mag Set"="Mag Set 2", "Gyro Set"="Gyro Set 2", "Fast"=TRUE, "CalSamples"=30 ("CalAvg"), "I2C Bus"=i2c_bus."I2C On-Board") -> ("AdaIMUDevRef Out"=w219:T7)  [unwired: 2 in, 2 out]
      n54 = call "IMURefNum Registry Set.vi"("refnum name"="AdaFruit IMU RefNum", "AdaIMUDevRef"=w219) -> ()  [unwired: 8 in, 2 out]
    }
    frame Enabled {
    }
  }
  n55 = Unbundle By Name("Mag Set") -> ("Sense Enable"=w50:bool, "Range"=w49:u8, "Data Rate"=w54:T18, "Mag Scale"=w46:T17, "Mag Offset"=w45:cluster{"Xzero":dbl, "Yzero":dbl, "Zzero":dbl}, "Anomaly Thresh"=w41:dbl, "Local Mag"=w40:dbl)
  n56 = case shown="True" w51 {
    tunnel: [u8 0 ("Device Address") w254] -> w52
    tunnel: w67 -> [_ w229]
    tunnel: w66 -> [_ w228]
    tunnel: w65 -> [_ w227]
    tunnel: w58 -> [_ w226]
    tunnel: "Controller" -> [_ w225]
    tunnel: "I2C Bus" -> [_ w224]
    frame False {
    }
    frame True {
      # "Accelerometer"
      n57 = call <vilib>:"WPI_I2COpen.vi"("Device Address"=u8 25 ("Data To Send"), "I2C Bus"=w224, "Controller"=w225) -> ("I2CDevRef"=w232:T9)  [unwired: 7 in, 1 out]
      n58 = Boolean To (0,1)(Boolean=w229) -> (0, 1=w253:i16)
      n59 = Logical Shift(y=i16 4, x=w228) -> (x << y=w249:u32)
      n60 = Logical Shift(y=i16 3, x=w253) -> (x << y=w250:i16)
      n61 = Or(x=w250, y=w249) -> (x .or. y?=w233:u32)
      n62 = Build Array(w233) -> (w235:u32[])
      n63 = call <vilib>:"WPI_I2CWrite.vi"("I2CDataToSend"=w235, "I2CRegister"=u8 33 ("Data To Send"), "I2CDevRef"=w232) -> ("I2CDevRef"=w231:T9)  [unwired: 7 in, 1 out]
      n64 = Logical Shift(y=i16 4, x=w226) -> (x << y=w238:u8)
      n65 = Or(x=u8 128 ("Data To Send"), y=w238) -> (x .or. y?=w237:u8)
      n66 = Build Array(w237) -> (w241:u8[])
      n67 = call <vilib>:"WPI_I2CWrite.vi"("I2CDataToSend"=w241, "I2CRegister"=u8 35 ("Data To Send"), "I2CDevRef"=w231) -> ("I2CDevRef"=w230:T9)  [unwired: 7 in, 1 out]
      n68 = Logical Shift(y=i16 4, x=w227) -> (x << y=w244:u32)
      n69 = Or(x=w244, y=u8 7 ("Data To Send")) -> (x .or. y?=w243:u32)
      n70 = Build Array(w243) -> (w247:u32[])
      n71 = call <vilib>:"WPI_I2CWrite.vi"("I2CDataToSend"=w247, "I2CRegister"=u8 32 ("Data To Send"), "I2CDevRef"=w230) -> ("I2CDevRef"=w242:T9)  [unwired: 7 in, 1 out]
      n72 = Unbundle By Name(w242) -> ("Device Address"=w254:u8)
    }
  }
  n73 = case shown="True" w50 {
    tunnel: "Controller" -> [_ w276]
    tunnel: w49 -> [_ w275]
    tunnel: [u8 0 ("Device Address") w274] -> w57
    tunnel: w54 -> [_ w259]
    tunnel: "I2C Bus" -> [_ w257]
    frame False {
    }
    frame True {
      # "Magnetometer"
      n74 = call <vilib>:"WPI_I2COpen.vi"("Device Address"=u8 30 ("Data To Send"), "I2C Bus"=w257, "Controller"=w276) -> ("I2CDevRef"=w271:T9)  [unwired: 7 in, 1 out]
      n75 = Logical Shift(y=i16 5, x=w275) -> (x << y=w261:u8)
      n76 = Build Array(w261) -> (w269:u8[])
      n77 = call <vilib>:"WPI_I2CWrite.vi"("I2CDataToSend"=w269, "I2CRegister"=u8 1 ("Data To Send"), "I2CDevRef"=w271) -> ("I2CDevRef"=w272:T9)  [unwired: 7 in, 1 out]
      n78 = Logical Shift(y=i16 2, x=w259) -> (x << y=w260:u32)
      n79 = Build Array(w260) -> (w266:u32[])
      n80 = call <vilib>:"WPI_I2CWrite.vi"("I2CDataToSend"=w266, "I2CRegister"=u8 0 ("Data To Send"), "I2CDevRef"=w272) -> ("I2CDevRef"=w273:T9)  [unwired: 7 in, 1 out]
      n81 = Build Array(i16 0 ("y")) -> (w264:i16[])
      n82 = call <vilib>:"WPI_I2CWrite.vi"("I2CDataToSend"=w264, "I2CRegister"=u8 2 ("Data To Send"), "I2CDevRef"=w273) -> ("I2CDevRef"=w265:T9)  [unwired: 7 in, 1 out]
      n83 = Unbundle By Name(w265) -> ("Device Address"=w274:u8)
    }
  }
  n84 = Bundle By Name(cluster=T7 {"DevStatus"={"status"=FALSE, "code"=0, "source"=""}, "Gyro Address"=0, "Gyro Range"=0, "Mean Rates"={"Xmo"=0.0, "Ymo"=0.0, "Zmo"=0.0}, "StdDev Rates"={"Xsdo"=0.0, "Ysdo"=0.0, "Zsdo"=0.0}, "Fast"=FALSE, "Reset"=FALSE, "Accel Address"=0, "Accel Range"=0, "Accel Scale"={"Xscale"=0.0, "Yscale"=0.0, "Zscale"=0.0}, "Mag Address"=0, "Mag Range"=0, "G Sense"=FALSE, "A Sense"=FALSE, "M Sense"=FALSE, "Accel Offset"={"Xzero"=0.0, "Yzero"=0.0, "Zzero"=0.0}, "Motion Thresh"=0.0, "Mag Scale"={"Xscale"=0.0, "Yscale"=0.0, "Zscale"=0.0}, "Mag Offset"={"Xzero"=0.0, "Yzero"=0.0, "Zzero"=0.0}, "I2C Bus"=enum."I2C On-Board", "Handle"=0, "Controller"=enum."Controller 1", "Anomaly Thresh"=0.0, "Local Mag"=0.0} ("AdaIMUDevRef"), "G Sense"=w53, "Gyro Range"=w63, "DevStatus"=w71, "Controller"=w42, "Gyro Address"=w70, "Handle"=w43, "I2C Bus"=w44, "Fast"="Fast", "A Sense"=w51, "Accel Address"=w52, "Accel Range"=w58, "Accel Scale"=w59, "Motion Thresh"=w56, "M Sense"=w50, "Mag Address"=w57, "Mag Range"=w49, "Mag Scale"=w46, "Mag Offset"=w45, "Anomaly Thresh"=w41, "Local Mag"=w40) -> (w37:T7)
  n85 = for {
    N: 8 -> [_]
    tunnel: w37 -> [w280]
    tunnel: w48 -> [w279]
    tunnel: [w278] -> w38
    tunnel: [w277] -> w47
    n86 = call "IMURead.vi"("AdaIMUDevRef"=w280, "error in"=w279) -> ("AdaIMUDevRef Out"=w278:T7, "error out"=w277:errorcluster)  [unwired: 9 in, 3 out]
    n87 = Wait (ms)(milliseconds to wait=u32 50) -> ()  [unwired: 1 out]
  }
  n88 = Initialize Array(0.0 ("element"), "CalSamples", 3 ("dimension size")) -> (w29:dbl[][])
  n89 = Initialize Array(0.0 ("element"), 3 ("dimension size")) -> (w11:dbl[])
  n90 = while "Gyro & Accelerometer Calibration" {
    tunnel: w38 -> [w304]
    tunnel: w47 -> [w317]
    tunnel: "CalSamples" -> [w312]
    tunnel: w29 -> [w311]
    tunnel: w29 -> [w307]
    tunnel: [w306] -> w22
    tunnel: [w302] -> w15
    tunnel: [w301] -> w14
    tunnel: w11 -> [w300]
    tunnel: [w284] -> w4
    tunnel: [w283] -> w3
    i -> [w282]
    stop <- w285 stop-if-true
    # "Preserve Mag Set\ncal values should\nMagnetic Cal be\nunrequested."
    # "'Zero' Gyro rate, Accelerometer,\nand Magnetometer biases\n(offsets).  Initialize Mag scale\nfactors to 1.  This allows the\nIMU Open VI to call the IMU\nRead VI and obtain raw readings\nso IMU Open can determine\ncalibration settings for the three\ndevices.\n\nNote: the Accelerometer scale\nfactors are not initialized since\nthat calibration should be\nperformed off robot, as it\nrequires the sensor to be moved\nin all 3 dimensions.  These values\nare either determined experimentally\noff-robot (to improve upon the\nstandard sensitivity values given in\nthe sensor spec sheet), or assumed\nto be a value of one for each axis."
    # "Report Bad Calibration if any\naxis Standard Deviation is too\nhigh.  This is caused by movement\nduring the cal period, insufficient\nwarmup time, or possibly bad\nsensor.  Thresholds were\ndetermined experimentally."
    # "If BadCal, try one\nmore time."
    # "Read a sample set of measurements\nfrom each axis for Gyro and Accelerometer\ncalibration.  Sample size determined by\nCalSamples parameter.  The intent is to\ndetermine the Gyro rate and Accelerometer\noutputs under the condition that the \nsensor is not moving, in order to identify\na 'zero' rate reference for the Gyro and the\nbiases (offsets from zero) for the Accel.\nMagnetometer calibration is performed next\n(if MagCal selected True), since this requires\nthe sensor to be moving as data is collected."
    # "Determine zero (rate) reference\n(dataset mean) for each axis, and\nevaluate level of variation\n(dataset standard deviation)\nto assess quality of calibration."
    n91 = flat-sequence {
      tunnel: w304 -> [w340]
      tunnel: [w340] -> w303
      tunnel: [w339] -> w302
      tunnel: [w338] -> w301
      tunnel: [w345] -> w305
      tunnel: w303 -> [w344]
      frame #0 {
        n92 = Unbundle By Name(w340) -> ("Mag Scale"=w339:T17, "Mag Offset"=w338:cluster{"Xzero":dbl, "Yzero":dbl, "Zzero":dbl})
      }
      frame #1 {
        w342 = T19 {"Accel Zero.Zzero"=0.0, "Accel Zero.Zzero 2"=0.0, "Accel Zero.Zzero 3"=0.0}
        n93 = Bundle By Name(cluster=w344, "Mean Rates"=w342, "Accel Offset"=T19 {"Accel Zero.Zzero"=0.0, "Accel Zero.Zzero 2"=0.0, "Accel Zero.Zzero 3"=1.0}, "Mag Offset"=w342, "Mag Scale"=T19 {"Accel Zero.Zzero"=1.0, "Accel Zero.Zzero 2"=1.0, "Accel Zero.Zzero 3"=1.0}) -> (w345:T7)
      }
    }
    n94 = node-c288(i64 30 ("Period"), 200 ("Priority")) -> (w337:T10)  [unwired: 1 in]
    n95 = timed-loop "Generate Accel & Gyro Dataset" {
      tunnel: w317 -> [w360]
      tunnel: w305 -> [w361]
      timing: w337 -> [_]
      timing-out: [_] -> w336
      tunnel: w311 -> [w357]
      tunnel: [w364] -> w331
      tunnel: [w366] -> w318
      tunnel: [w365] -> w335
      tunnel: w312 -> [w362]
      tunnel: [w356] -> w292
      tunnel: w307 -> [w355]
      tunnel: w300 -> [w352]
      i -> [w346]
      stop <- w367 stop-if-true
      n96 = Decrement(x=w362) -> (x-1=w359:i32)
      n97 = call "IMURead.vi"("AdaIMUDevRef"=w361, "error in"=w360) -> ("AdaIMUDevRef Out"=w366:T7, "Gyro"=w354:T13, "Accel"=w348:T14, "error out"=w365:errorcluster)  [unwired: 9 in, 1 out]
      n98 = Equal?(x=w359, y=w346) -> (x = y?=w367:bool)
      n99 = Unbundle By Name(w348) -> ("Xaccel"=w350:dbl, "Yaccel"=w349:dbl, "Zaccel"=w347:dbl)
      n100 = Cluster To Array(cluster=w354) -> (array=w353:dbl[])
      n101 = Replace Array Subset(array=w352, new element #1=w350, new element #2=w349, new element #3=w347) -> (w351:dbl[])  [unwired: 3 in]
      n102 = feedback #1(w357) -> (w363:dbl[][])
      n103 = Replace Array Subset(array=w363, new element=w353, index (row)=w346) -> (w364:dbl[][])  [unwired: 1 in]
      n104 = feedback-in #1(w364) -> ()
      n105 = feedback #2(w355) -> (w358:dbl[][])
      n106 = Replace Array Subset(array=w358, new element=w351, index (row)=w346) -> (w356:dbl[][])  [unwired: 1 in]
      n107 = feedback-in #2(w356) -> ()
    }
    "error out" <- w335
    n108 = node-c288(w336) -> ()  [unwired: 1 out]
    n109 = Index Array(array=w292, index (col)=0 ("index")) -> (element=w293:dbl[])  [unwired: 1 in]
    n110 = Index Array(array=w292, index (col)=1 ("index")) -> (element=w294:dbl[])  [unwired: 1 in]
    n111 = Index Array(array=w292, index (col)=2 ("index")) -> (element=w295:dbl[])  [unwired: 1 in]
    n112 = call <vilib>:"Std Deviation and Variance.vi"("X"=w293) -> ("mean"=w291:dbl, "standard deviation"=w288:dbl)  [unwired: 1 in, 1 out]
    n113 = call <vilib>:"Std Deviation and Variance.vi"("X"=w294) -> ("mean"=w290:dbl, "standard deviation"=w287:dbl)  [unwired: 1 in, 1 out]
    n114 = call <vilib>:"Std Deviation and Variance.vi"("X"=w295) -> ("mean"=w289:dbl, "standard deviation"=w286:dbl)  [unwired: 1 in, 1 out]
    n115 = Index Array(array=w331, index (col)=0 ("index")) -> (element=w334:dbl[])  [unwired: 1 in]
    n116 = Index Array(array=w331, index (col)=1 ("index")) -> (element=w333:dbl[])  [unwired: 1 in]
    n117 = Index Array(array=w331, index (col)=2 ("index")) -> (element=w332:dbl[])  [unwired: 1 in]
    n118 = call <vilib>:"Std Deviation and Variance.vi"("X"=w334) -> ("mean"=w326:dbl, "standard deviation"=w322:dbl)  [unwired: 1 in, 1 out]
    n119 = call <vilib>:"Std Deviation and Variance.vi"("X"=w333) -> ("mean"=w325:dbl, "standard deviation"=w299:dbl)  [unwired: 1 in, 1 out]
    n120 = call <vilib>:"Std Deviation and Variance.vi"("X"=w332) -> ("mean"=w324:dbl, "standard deviation"=w321:dbl)  [unwired: 1 in, 1 out]
    n121 = Max & Min(x=w287, y=w286) -> (max(x,y)=w308:dbl)  [unwired: 1 out]
    n122 = Max & Min(x=w288, y=w308) -> (max(x,y)=w309:dbl)  [unwired: 1 out]
    n123 = Greater?(x=w309, y=0.03) -> (0:w283:bool)
    n124 = Max & Min(x=w299, y=w321) -> (max(x,y)=w323:dbl)  [unwired: 1 out]
    n125 = Max & Min(x=w322, y=w323) -> (max(x,y)=w320:dbl)  [unwired: 1 out]
    n126 = Bundle By Name(cluster=w318, "Mean Rates.Xmo"=w326, "StdDev Rates.Xsdo"=w322, "Mean Rates.Ymo"=w325, "StdDev Rates.Ysdo"=w299, "Mean Rates.Zmo"=w324, "StdDev Rates.Zsdo"=w321, "Accel Offset.Xzero"=w291, "Accel Offset.Yzero"=w290, "Accel Offset.Zzero"=w289) -> (w306:T7)
    n127 = Greater?(x=w320, y=0.5) -> (0:w284:bool)
    n128 = Equal?(x=1, y=w282) -> (x = y?=w316:bool)
    n129 = Not(x=w284) -> (.not. x?=w314:bool)
    n130 = Or(x=w314, y=w316) -> (x .or. y?=w285:bool)
  }
  n131 = Bundle By Name(cluster=T1 {"BadCal Gyro"=FALSE, "BadCal Accel"=FALSE, "BadCal Mag"=FALSE} ("Cal Status"), "BadCal Gyro"=w4, "BadCal Accel"=w3) -> (w1:T1)
  n132 = case shown="True" "MagCal" {
    selector: "MagCal" -> [w376 w379]
    tunnel: [w376 w379] -> w19
    tunnel: [w377 w381] -> w21
    tunnel: w22 -> [w377 w381]
    frame False {
      n133 = local write "stop loop"(TRUE ("true")) -> ()
    }
    frame True {
      n134 = One Button Dialog(message="Rotate robot 360 deg in horizontal plane.\nBest data results from rotating about \nactual sensor axis.\n\nSelect OK to begin data collection.") -> ()  [unwired: 1 in, 1 out]
      "stop loop" <- FALSE ("true")
    }
  }
  n135 = case shown="True" w19 {
    frame False {
    }
    frame True {
      n136 = One Button Dialog(message="Select OK when\nrotation is complete.") -> (true=w382:bool)  [unwired: 1 in]
      n137 = local write "stop loop"(w382) -> ()
    }
  }
  n138 = node-c288(i64 30 ("Period"), 200 ("Priority")) -> (w34:T10)  [unwired: 1 in]
  n139 = Initialize Array(0.0 ("element"), 3 ("dimension size")) -> (w8:dbl[])
  n140 = Initialize Array(0.0 ("element"), 0 ("Samples"), 3 ("dimension size")) -> (w24:dbl[][])
  n141 = timed-loop "Generate Magnetometer Dataset" {
    timing: w34 -> [_]
    timing-out: [_] -> w33
    tunnel: [w391] -> w17
    tunnel: [w389] -> w18
    tunnel: w24 -> [w388]
    tunnel: w19 -> [w386]
    tunnel: w21 -> [w387]
    tunnel: [w386] -> w16
    tunnel: w8 -> [w384]
    i -> [w390]
    stop <- w385 stop-if-true
    # "Gather Mag data as Robot is rotated in X-Y plane."
    n142 = local read "stop loop"() -> (w385:bool)
    n143 = case shown="True" w386 {
      tunnel: [w393 w405] -> w391
      tunnel: w390 -> [_ w403]
      tunnel: [w392 w402] -> w389
      tunnel: w388 -> [w392 w401]
      tunnel: w387 -> [w393 w400]
      tunnel: w384 -> [_ w395]
      frame False {
      }
      frame True {
        n144 = call "IMURead.vi"("AdaIMUDevRef"=w400) -> ("AdaIMUDevRef Out"=w405:T7, "Mag"=w398:T15)  [unwired: 10 in, 3 out]
        n145 = Unbundle By Name(w398) -> ("Xmag"=w397:dbl, "Ymag"=w399:dbl, "Zmag"=w396:dbl)
        n146 = Replace Array Subset(array=w395, new element #1=w397, new element #2=w399, new element #3=w396) -> (w394:dbl[])  [unwired: 3 in]
        n147 = feedback #3(w401) -> (w404:dbl[][])
        n148 = Insert Into Array(array=w404, index (row)=w403, new element=w394) -> (w402:dbl[][])  [unwired: 1 in]
        n149 = feedback-in #3(w402) -> ()
      }
    }
  }
  n150 = node-c288(w33) -> ()  [unwired: 1 out]
  n151 = case "Magnetometer Calibration" shown="True" w16 {
    tunnel: w18 -> [_ w440]
    tunnel: w17 -> [w412 w446]
    tunnel: [w411 w445] -> w7
    tunnel: w15 -> [w410 _]
    tunnel: w14 -> [w409 _]
    tunnel: [FALSE w418] -> w5
    frame False {
      # "If not calibrating Magnetometer, use calibration settings\nprovided to IMU Open within Mag Set cluster."
      n152 = Bundle By Name(cluster=w412, "Mag Scale"=w410, "Mag Offset"=w409) -> (w411:T7)
    }
    frame True {
      (unwired) path "C:/tmp/Mag_data.csv" ("file path (dialog if empty)")
      w450 = 1.0 ("y")
      w447 = 2.0 ("y")
      # "Biaxial"
      # "Triaxial"
      # "cRIO address format"
      # "Store mag data to roboRIO for review"
      # "Report Bad Calibration if any magnetic\nvector magnitude is too different from\nEarth field.  This is caused by on-Robot\nSoft Iron, near-by off-Robot Hard Iron,\nor possibly bad sensor.  Threshold was\ndetermined experimentally."
      # "Z values"
      # "Y values"
      # "X values"
      # "Ref http://www.cypress.com/?docID=49962\neqs 38-43 (and correcting for typo in eq 43)\nfor simple calibration of Magnetometer\n(in 2D X-Y plane only)."
      n153 = Index Array(array=w440, index (col)=0 ("index (row)")) -> (element=w431:dbl[])  [unwired: 1 in]
      n154 = Index Array(array=w440, index (col)=1 ("index (row)")) -> (element=w430:dbl[])  [unwired: 1 in]
      n155 = Bundle(w431, w430) -> (→"XY Mag":cluster{dbl[], dbl[]})  [unwired: 1 in]
      n156 = call-poly <vilib>:"Write To Spreadsheet File.vi"("delimiter (\\t)"="," ("delimiter (\\t)"), "2D data"=w440, "file path (dialog if empty)"=path "/home/lvuser/Mag_data.csv") -> ()  [unwired: 5 in, 1 out]
      n157 = Index Array(array=w440, index (col)=2 ("index (row)")) -> (element=w429:dbl[])  [unwired: 1 in]
      n158 = Array Max & Min(array=w431) -> (max value=w456:dbl, min value=w455:dbl)  [unwired: 2 out]
      n159 = Array Max & Min(array=w430) -> (max value=w459:dbl, min value=w458:dbl)  [unwired: 2 out]
      n160 = Add(x=w456, y=w455) -> (x+y=w457:dbl)
      n161 = Subtract(x=w456, y=w455) -> (x-y=w453:dbl)
      n162 = Add(x=w459, y=w458) -> (x+y=w460:dbl)
      n163 = Subtract(x=w459, y=w458) -> (x-y=w454:dbl)
      n164 = Divide(x=w457, y=w447) -> (x/y=w449:dbl)
      n165 = Divide(x=w460, y=w447) -> (x/y=w448:dbl)
      n166 = Divide(x=w454, y=w453) -> (x/y=w452:dbl)
      n167 = Reciprocal(x=w452) -> (1/x=w451:dbl)
      n168 = Max & Min(x=w452, y=w450) -> (max(x,y)=w425:dbl)  [unwired: 1 out]
      "Xmagscale" <- w425
      n169 = Max & Min(x=w450, y=w451) -> (max(x,y)=w428:dbl)  [unwired: 1 out]
      "Ymagscale" <- w428
      n170 = Multiply(x=w449, y=w425) -> (x*y=w427:dbl)
      "Xmagzero" <- w427
      n171 = Multiply(x=w448, y=w428) -> (x*y=w426:dbl)
      "Ymagzero" <- w426
      n172 = Array Size(array=w431) -> (size(s)=w439:i32)
      n173 = for {
        N: w439 -> [_]
        tunnel: w431 -> [w470] mode=indexing
        tunnel: w430 -> [w467] mode=indexing
        tunnel: w429 -> [w478] mode=indexing
        tunnel: [w477] -> w438 mode=indexing
        tunnel: [w473] -> w417 mode=indexing
        tunnel: w425 -> [w471]
        tunnel: w428 -> [w466]
        tunnel: w427 -> [w469]
        tunnel: w426 -> [w465]
        tunnel: [w464] -> w422 mode=indexing
        tunnel: [w463] -> w421 mode=indexing
        # "Root-Sum-Square"
        n174 = Multiply(x=w470, y=w471) -> (x*y=w472:dbl)
        n175 = Multiply(x=w467, y=w466) -> (x*y=w468:dbl)
        n176 = Subtract(x=w472, y=w469) -> (x-y=w464:dbl)
        n177 = Subtract(x=w468, y=w465) -> (x-y=w463:dbl)
        n178 = Square(x=w470) -> (x^2=w479:dbl)
        n179 = Square(x=w467) -> (x^2=w480:dbl)
        n180 = Square(x=w478) -> (x^2=w481:dbl)
        n181 = Square(x=w464) -> (x^2=w476:dbl)
        n182 = Square(x=w463) -> (x^2=w475:dbl)
        n183 = Compound Arithmetic op=ADD(w479, w480, w481) -> (w482:dbl)
        n184 = Compound Arithmetic op=ADD(w476, w475) -> (w474:dbl)
        n185 = Square Root(x=w482) -> (sqrt(x)=w477:dbl)
        n186 = Square Root(x=w474) -> (sqrt(x)=w473:dbl)
      }
      n187 = Bundle By Name(cluster=w446, "Mag Offset.Xzero"=w427, "Mag Offset.Yzero"=w426, "Mag Offset.Zzero"=0.0, "Mag Scale.Xscale"=w425, "Mag Scale.Yscale"=w428, "Mag Scale.Zscale"=1.0) -> (w445:T7)
      n188 = Array Max & Min(array=w438) -> (max value=w437:dbl, min value=w433:dbl)  [unwired: 2 out]
      n189 = call <vilib>:"Std Deviation and Variance.vi"("X"=w417) -> ("mean"=→"Local Magnitude (uT)":dbl, "standard deviation"=w415:dbl)  [unwired: 1 in, 1 out]
      n190 = Bundle(w422, w421) -> (→"XY Mag, Cal'd":cluster{dbl[], dbl[]})  [unwired: 1 in]
      n191 = Subtract(x=w437, y=w433) -> (x-y=w436:dbl)
      n192 = Multiply(x=w415, y=3.0) -> (x*y=w413:dbl)
      "Anomaly Tol (uT)" <- w413
      n193 = Divide(x=w436, y=2.0) -> (x/y=w434:dbl)
      "Half-Range" <- w434
      n194 = Greater?(x=w413, y=4.0) -> (0:w418:bool)
      n195 = Add(x=w434, y=w433) -> (x+y=→"Mid-Pnt":dbl)
    }
  }
  "AdaIMUDevRef Out" <- w7
  n196 = Bundle By Name(cluster=w1, "BadCal Mag"=w5) -> (→"Cal Result":T1)
